vi "New Image Rotate.vi"(8 "error in (no error)":errorcluster, 10 "Image":T1, 11 "Rotate in":refnum<class "Rotate.lvclass">) -> (0 "error out":errorcluster, 3 "Rotate out":refnum<class "Rotate.lvclass">)   [LabVIEW 2016, in "Rotate.lvclass"]
uses:
  Rotation/Rotate.lvclass
  <vilib>/vision/Image Controls.llb/IMAQ Image.ctl
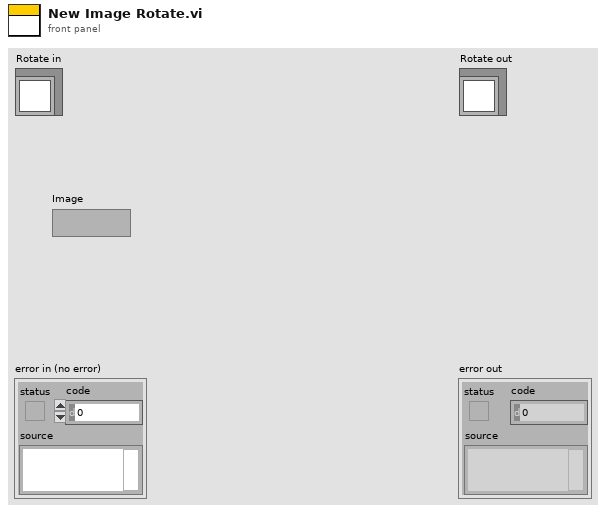
[diagram p1: front panel]
types:
  T1 = typedef "IMAQ Image.ctl" = refnum<image>
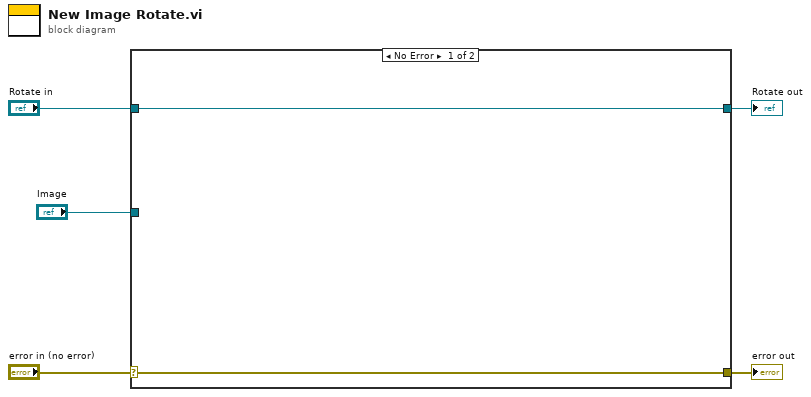
[diagram p0: block diagram]
diagram:
  n1 = case shown="No Error" "error in (no error)" {
    selector: "error in (no error)" -> [w6 w9]
    tunnel: [w6 w9] -> w4
    tunnel: [w7 w8] -> w2
    tunnel: "Rotate in" -> [w7 w8]
    tunnel: "Image" -> [_ _]
    frame No Error {
    }
    frame Error {
    }
  }
  "error out" <- w4
  "Rotate out" <- w2
